vi "WFCompose_WFpadOrTrim.vi"(10 "Duration (s)":dbl min=0.0, 11 "Waveform In":waveform(dbl)={"t0"=timestamp(0 s since 1904-01-01), "dt"=0.0, "Y"=[]}) -> (3 "Analog Waveform Out":waveform(dbl))   [LabVIEW 2013]
uses:
  <vilib>/Waveform/WDTOps.llb/WDT Waveform Duration DBL.vi
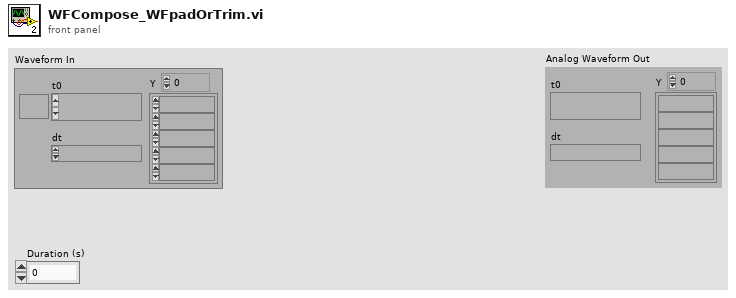
[diagram p1: front panel]
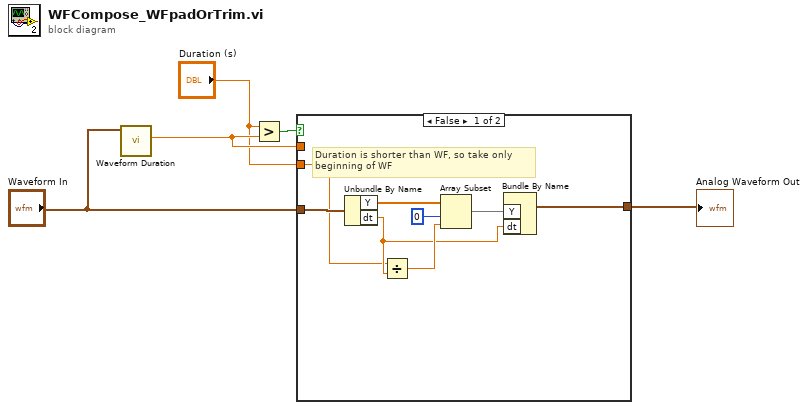
[diagram p0: block diagram]
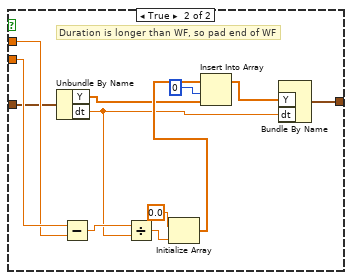
[diagram p2: hidden frame]
diagram:
  n1 = call-poly <vilib>:"Waveform Duration.vi"("waveform in"="Waveform In") -> ("duration"=w4:dbl)  [unwired: 8 in, 2 out]
  n2 = Greater?(x="Duration (s)", y=w4) -> (0:w5:bool)
  n3 = case shown="False" w5 {
    tunnel: "Waveform In" -> [w13 w20]
    tunnel: "Duration (s)" -> [w7 w25]
    tunnel: w4 -> [_ w24]
    tunnel: [w6 w19] -> w1
    frame False {
      # "Duration is shorter than WF, so take only beginning of WF"
      n4 = Unbundle By Name(w13) -> ("Y"=w12:dbl[], "dt"=w8:dbl)
      n5 = Divide(x=w7, y=w8) -> (x/y=w10:dbl)
      n6 = Array Subset(array=w12, index=0, length=w10) -> (w9:dbl[])
      n7 = Bundle By Name("Y"=w9, "dt"=w8) -> (w6:waveform(dbl))  [unwired: 1 in]
    }
    frame True {
      # "Duration is longer than WF, so pad end of WF"
      n8 = Unbundle By Name(w20) -> ("Y"=w16:dbl[], "dt"=w14:dbl)
      n9 = Subtract(x=w25, y=w24) -> (x-y=w23:dbl)
      n10 = Divide(x=w23, y=w14) -> (x/y=w22:dbl)
      n11 = Initialize Array(0.0 ("element"), w22) -> (w18:dbl[])
      n12 = Insert Into Array(array=w18, index=0, new element=w16) -> (w15:dbl[])
      n13 = Bundle By Name("Y"=w15, "dt"=w14) -> (w19:waveform(dbl))  [unwired: 1 in]
    }
  }
  "Analog Waveform Out" <- w1
